vi "Update Controller.vi"(8 "error in":errorcluster, 11 "Humidity Control in":refnum<class "Humidity Control.lvclass">) -> (0 "error out":errorcluster, 3 "Humidity Control out":refnum<class "Humidity Control.lvclass">)   [LabVIEW 2015, in "Humidity Control.lvclass"]
doc: "Providing the correct RH and the setpoint, update the controller such that it provides the proper response."
uses:
  Humidity Control.lvclass
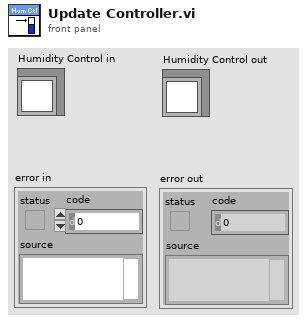
[diagram p1: front panel]
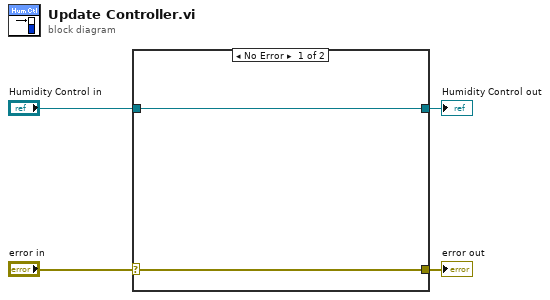
[diagram p0: block diagram]
diagram:
  n1 = case shown="No Error" "error in" {
    selector: "error in" -> [w6 w8]
    tunnel: [w6 w8] -> w3
    tunnel: [w5 w7] -> w1
    tunnel: "Humidity Control in" -> [w5 w7]
    frame No Error {
    }
    frame Error {
    }
  }
  "error out" <- w3
  "Humidity Control out" <- w1
